vi "Generate Wavforms.vi"(1 "Sounds.lvclass":refnum<class "Sound.lvclass">) -> (0 "Array":waveform(dbl)[](array[waveform]))   [LabVIEW 2017, in "Sound.lvclass"]
doc: "This method creates a waveform fo the sound to be played. This method MUST be overridend by children of sound."
uses:
  Sound.lvclass
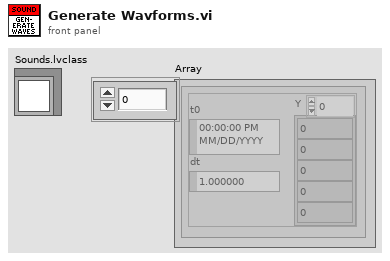
[diagram p1: front panel]
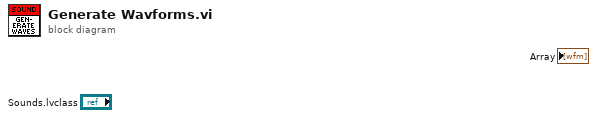
[diagram p0: block diagram]
diagram:
